vi "Host_FormatUDP.vi"() -> (3 "data string":string)   [LabVIEW 2018]
doc: "Formats the string to be sent to SpaceX via UDP.\nPulls in sensor data and translates them into metric and their respective data types."
uses:
  Master/DAQ/Master_DataControl.ctl
  Master/DAQ/TypeDef_cRIOData.ctl
  Master/IMU/TypeDef_IMUData.ctl
  Master/CAN/TypeDef_BMSData.ctl
  Master/CAN/TypeDef_BMS_Status.ctl
  Master/CAN/MotorController/fixedMotorData.ctl
  Master/CAN/MotorController/Type_Def MotorStatus.ctl
  Type_Def/Type_Def ControlState.ctl
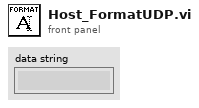
[diagram p1: front panel]
types:
  T1 = typedef "Master_DataControl.ctl" = cluster{"cRIO Data":T2, "IMU Data":T3, "BMS Data":T4, "Motor Data":T6}
  T2 = typedef "TypeDef_cRIOData.ctl" = cluster{"Time (ms)":dbl, "24V Battery (V)":dbl, "LowV Current (A)":dbl, "Fiducial Sensor (V)":dbl, "PV Pressure (psig)":dbl, "Flow Sensor (V)":dbl, "Temp Fairing (F)":dbl, "Temp Reservoir (F)":dbl, "HallEffect Right (in)":dbl, "HallEffect Left (in)":dbl, "PT Tank (psig)":dbl, "PT Clamp Right (psig)":dbl, "PT Clamp Left (psig)":dbl, "PT Brake (psig)":dbl, "PT Cooling (psig)":dbl, "Displacement (ft)":dbl, "Velocity (ft/s)":dbl}
  T3 = typedef "TypeDef_IMUData.ctl" = cluster{"x acceleration (g)":dbl, "Pressure (psia)":dbl, "Temperature (F)":dbl}
  T4 = typedef "TypeDef_BMSData.ctl" = cluster{"Max Cell Voltage (V)":dbl, "Max Cell ID":dbl, "Min Cell Voltage (V)":dbl, "Min Cell ID":dbl, "State of Charge (%)":dbl, "Average Voltage (V)":dbl, "Voltage Delta (V)":dbl, "Pack Current (A)":dbl, "Pack Voltage (V)":dbl, "Max Resistance (Ohm)":dbl, "Min Resistance (Ohm)":dbl, "Average Resistance (Ohm)":dbl, "Delta Resistance (Ohm)":dbl, "Highest Temperature(F)":dbl, "BmsStatus":T5}
  T5 = typedef "TypeDef_BMS_Status.ctl" = cluster{"isFault":bool, "isolationMonitoring":bool}
  T6 = typedef "fixedMotorData.ctl" = cluster{"Velo (RPM)":dbl, "MotorTemp(F)":dbl, "CtrlTemp(F)":dbl, "DcLinkVolt(V)":dbl, "ErrorCode":dbl, "motorStatus":T7, "isAlive":bool, "motorControllerState":u16}
  T7 = typedef "Type_Def MotorStatus.ctl" = cluster{"isReady":bool, "isOn":bool, "isOperEn":bool, "isFault":bool, "isVoltEn":bool, "targetReached":bool, "isWarning":bool}
  T8 = typedef "Type_Def ControlState.ctl" = enum16{"Blank", "Systems Check", "Idle", "Ready", "Pushing", "CrawlingPrecharge", "Braking", "Fault", "Boot Up", "Unpowered", "Crawling", "Shutdown", "Service Push", "Service Wait", "Vent", "Precharge"}
  T9 = cluster{"Team ID":u8, u8, i32, i32, i32, i32, i32, i32, i32, u32}
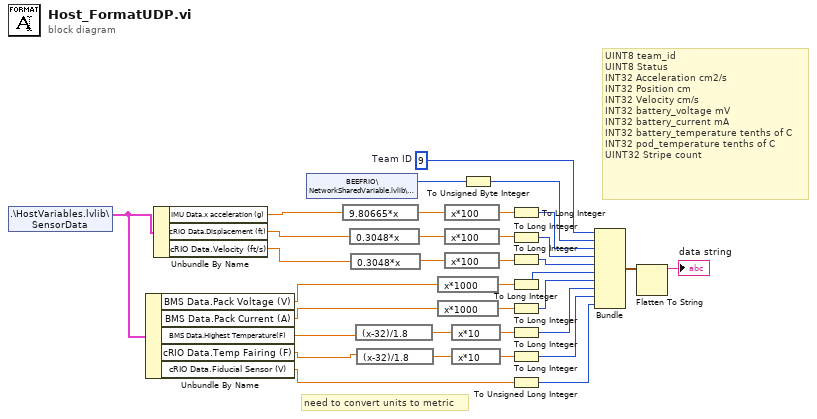
[diagram p0: block diagram]
diagram:
  w18 = u8 9  # Team ID
  # "need to convert units to metric"
  # "UINT8 team_id\nUINT8 Status\nINT32 Acceleration cm2/s\nINT32 Position cm\nINT32 Velocity cm/s\nINT32 battery_voltage mV\nINT32 battery_current mA\nINT32 battery_temperature tenths of C\nINT32 pod_temperature tenths of C\nUINT32 Stripe count"
  n1 = shared-variable ".\\HostVariables.lvlib\\SensorData"() -> (w13:T1)  [unwired: 1 in, 1 out]
  n2 = Unbundle By Name(w13) -> ("BMS Data.Pack Voltage (V)"=w5:dbl, "BMS Data.Pack Current (A)"=w6:dbl, "BMS Data.Highest Temperature(F)"=w9:dbl, "cRIO Data.Temp Fairing (F)"=w8:dbl, "cRIO Data.Fiducial Sensor (V)"=w11:dbl)
  n3 = Unbundle By Name(w13) -> ("IMU Data.x acceleration (g)"=w15:dbl, "cRIO Data.Displacement (ft)"=w2:dbl, "cRIO Data.Velocity (ft/s)"=w1:dbl)
  n4 = shared-variable "BEEFRIO\\NetworkSharedVariable.lvlib\\CurrentState"() -> (w16:T8)  [unwired: 1 in, 1 out]
  n5 = expression code="9.80665*x"(w15) -> (w14:dbl)
  n6 = expression code="0.3048*x"(w2) -> (w4:dbl)
  n7 = expression code="0.3048*x"(w1) -> (w3:dbl)
  n8 = expression code="(x-32)/1.8"(w9) -> (w7:dbl)
  n9 = expression code="(x-32)/1.8"(w8) -> (w10:dbl)
  n10 = expression code="x*1000"(w5) -> (w26:dbl)
  n11 = expression code="x*1000"(w6) -> (w28:dbl)
  n12 = expression code="x*100"(w14) -> (w21:dbl)
  n13 = expression code="x*100"(w4) -> (w22:dbl)
  n14 = expression code="x*100"(w3) -> (w24:dbl)
  n15 = expression code="x*10"(w7) -> (w30:dbl)
  n16 = expression code="x*10"(w10) -> (w32:dbl)
  n17 = To Unsigned Byte Integer(number=w16) -> (unsigned 8bit integer=w12:u8)
  n18 = To Long Integer(number=w21) -> (32bit integer=w20:i32)
  n19 = To Long Integer(number=w22) -> (32bit integer=w23:i32)
  n20 = To Long Integer(number=w24) -> (32bit integer=w25:i32)
  n21 = To Long Integer(number=w26) -> (32bit integer=w27:i32)
  n22 = To Long Integer(number=w28) -> (32bit integer=w29:i32)
  n23 = To Long Integer(number=w30) -> (32bit integer=w31:i32)
  n24 = To Long Integer(number=w32) -> (32bit integer=w33:i32)
  n25 = To Unsigned Long Integer(number=w11) -> (unsigned 32bit integer=w34:u32)
  n26 = Bundle("Team ID"=w18, w12, w20, w23, w25, w27, w29, w31, w33, w34) -> (w19:T9)  [unwired: 1 in]
  n27 = Flatten To String(anything=w19) -> (data string=→"data string":string)  [unwired: 3 in, 2 out]
